vi "monitor_wm2.vi"() -> ()   [LabVIEW 2012]
panel:
  out "Orange":dbl(graph)=487.9912679215464
  out "Orange":dbl=487.9912679215464 format="%#_9g"
  in  "Orange Approx freq":dbl=488.0
  in  "Orange Channel":i32=15
  out "Ultra Blue":dbl(graph)=665.1601258342241
  out "Ultra Blue":dbl=665.1601258342241 format="%#_9g"
  in  "Ultra Blue Approx freq":dbl=665.2
  in  "Ultra Blue Channel":i32=10
  out "791":dbl(graph)=378.8378422550617
  out "Blue 2":dbl=303.7143863412696 format="%#_10g"
  out "Red 2":dbl=461.313111574132 format="%#_10g"
  in  "Blue approx freq":dbl=303.7
  in  "Red approx freq":dbl=461.3
  in  "791 Approx freq":dbl=378.8
  out "791 Frequency":dbl=378.8378422550617 format="%#_9g"
  in  "791 Channel":i32=6
  out "Current\nChannel":i32=13
  in  "Blue Channel":i32=12
  out "Blue":dbl(graph)=303.7143863412696
  in  "Red Channel":i32=2
  out "Red":dbl(graph)=461.313111574132
  in  "stop":bool
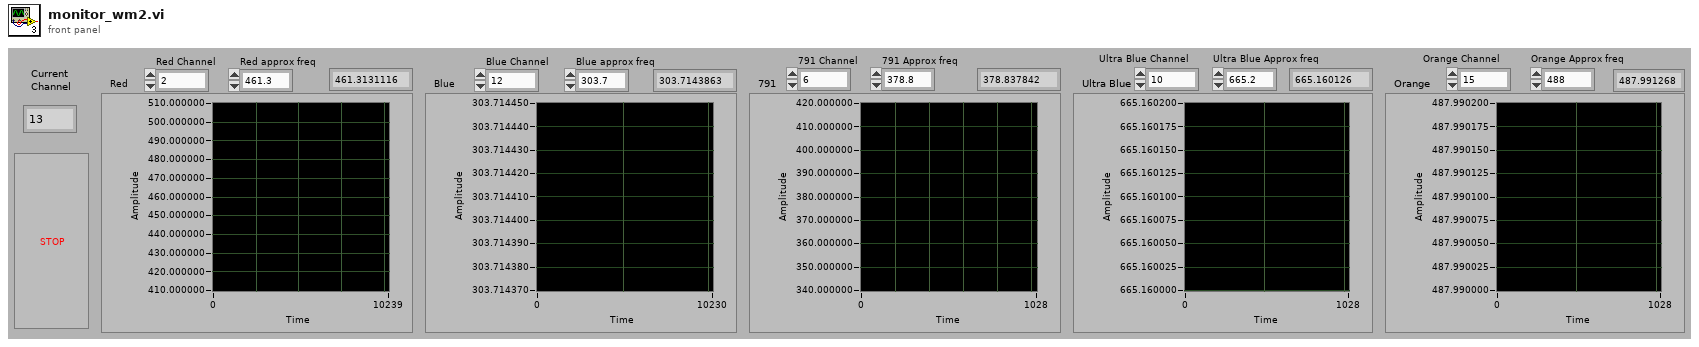
[diagram p1: front panel]
types:
  T1 = enum16{"Read", "Write", "ReadWrite", "BufferedRead", "BufferedReadWrite"}
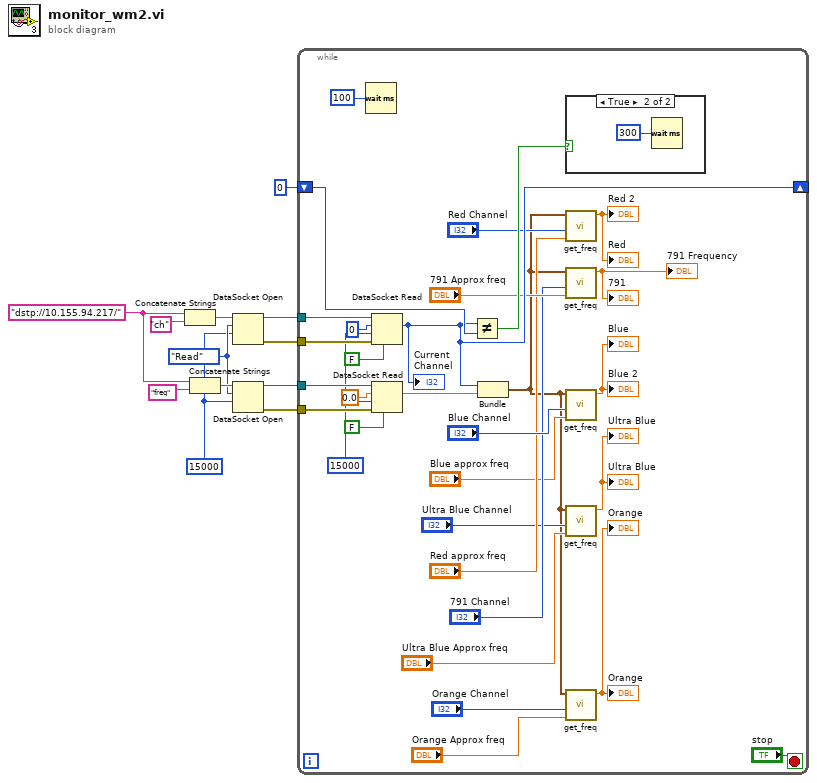
[diagram p0: block diagram]
diagram:
  w1 = 15000
  w7 = T1."Read" ("mode")
  w8 = "dstp://10.155.94.217/" ("string")
  n1 = Concatenate Strings(w8, "ch" ("string")) -> (w9:string)
  n2 = Concatenate Strings(w8, "freq" ("string")) -> (w10:string)
  n3 = DataSocket Open(9:w1, 10:w7, 11:w9) -> (0:w4:errorcluster, 3:w5:refnum<k13>)  [unwired: 1 in]
  n4 = DataSocket Open(9:w1, 10:w7, 11:w10) -> (0:w3:errorcluster, 3:w6:refnum<k13>)  [unwired: 1 in]
  n5 = while {
    tunnel: w6 -> [w38]
    tunnel: w5 -> [w37]
    tunnel: w4 -> [w36]
    tunnel: w3 -> [w35]
    shift-right: [w31] -> _
    shift-left: 0 ("Cur Ch") -> [w32]
    stop <- "stop" stop-if-true
    w13 = 15000
    n6 = Wait (ms)(milliseconds to wait=u32 100) -> ()  [unwired: 1 out]
    n7 = DataSocket Read(6:FALSE ("wait for updated value (T)"), 8:w36, 9:w13, 10:0 ("Cur Ch"), 11:w37) -> (2:w31:i32)  [unwired: 6 out]
    "Current\nChannel" <- w31
    n8 = DataSocket Read(6:FALSE ("wait for updated value (T)"), 8:w35, 9:w13, 10:0.0 ("Frequency"), 11:w38) -> (2:w30:dbl)  [unwired: 6 out]
    n9 = Not Equal?(x=w31, y=w32) -> (x != y?=w33:bool)
    n10 = Bundle("Cur Ch"=w31, "Frequency"=w30) -> (w15:cluster{"Cur Ch":i32, "Frequency":dbl})  [unwired: 1 in]
    n11 = case shown="True" w33 {
      frame False {
      }
      frame True {
        n12 = Wait (ms)(milliseconds to wait=u32 300) -> ()  [unwired: 1 out]
      }
    }
    n13 = call "get_freq.vi"("approx freq"="Red approx freq", "ch to get"="Red Channel", "wavemeter cluster"=w15) -> ("Frequency"=→"Red" →"Red 2":dbl)  [unwired: 8 in]
    n14 = call "get_freq.vi"("approx freq"="791 Approx freq", "ch to get"="791 Channel", "wavemeter cluster"=w15) -> ("Frequency"=→"791 Frequency" →"791":dbl)  [unwired: 8 in]
    n15 = call "get_freq.vi"("approx freq"="Blue approx freq", "ch to get"="Blue Channel", "wavemeter cluster"=w15) -> ("Frequency"=→"Blue" →"Blue 2":dbl)  [unwired: 8 in]
    n16 = call "get_freq.vi"("approx freq"="Ultra Blue Approx freq", "ch to get"="Ultra Blue Channel", "wavemeter cluster"=w15) -> ("Frequency"=→"Ultra Blue" →"Ultra Blue":dbl)  [unwired: 8 in]
    n17 = call "get_freq.vi"("approx freq"="Orange Approx freq", "ch to get"="Orange Channel", "wavemeter cluster"=w15) -> ("Frequency"=→"Orange" →"Orange":dbl)  [unwired: 8 in]
  }
